vi "display loop.vi"(0 "display queues":T4, 1 "sample length":i32=5000, 2 "reset":bool, 3 "time range (s)":dbl=2.2 format="%#_13g", 4 "mag type":enum16{"absolute", "relative"}(ring), 5 "volt slope":bool, 7 "error in":errorcluster, 8 "trigger":bool, 9 "hysteresis":dbl=0.1 format="%#_13g", 10 "disk queues":T4, 12 "gain":dbl=1.0) -> (11 "voltage slope":dbl, 13 "slope graphs":cluster{dbl[], dbl[]}[](array[cluster]), 14 "lifetime":dbl, 16 "magnet vs time":cluster{dbl[], dbl[]}[](array[cluster]), 17 "mag pos axes limits":cluster{"mag pos max":dbl, "mag pos min":dbl}, 18 "voltage axes":T1, 19 "crossing stats":T2, 20 "fit parameters":cluster{"a":dbl, "b":dbl, "theta":dbl, "b0":dbl}, 21 "angle":dbl, 22 "deg/hr":dbl format="%0.2f", 23 "pulse statistics":T3, 24 "angle graph":cluster{dbl[], dbl[]}[](array[cluster]), 25 "voltage graphs":cluster{dbl[], dbl[]}[](array[cluster]), 26 "magnet graphs":T6(array[cluster]), 27 "error out":errorcluster)   [LabVIEW 2017]
uses:
  typedefs/queue cluster.ctl
  typedefs/reading queue.ctl
  typedefs/reading.ctl
  typedefs/readingType.ctl
  typedefs/reading1.ctl
panel:
  in  "hrs":bool=TRUE
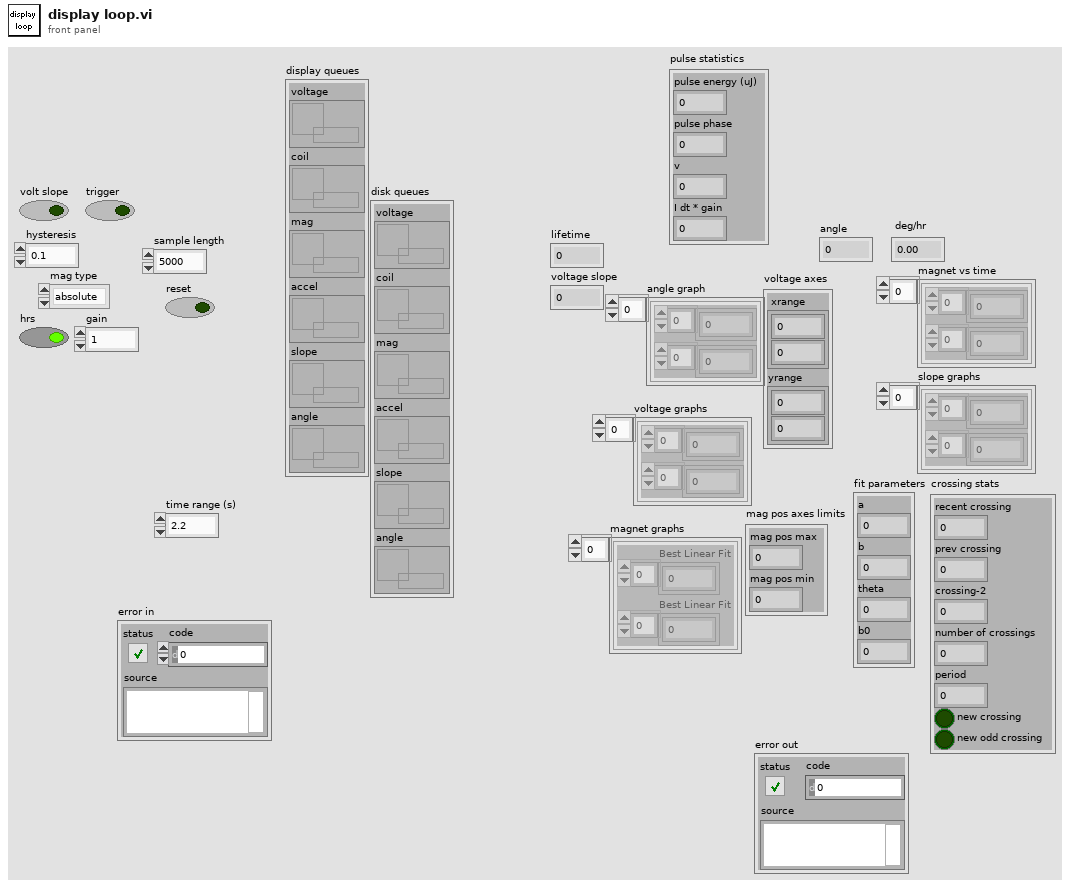
[diagram p1: front panel]
types:
  T1 = cluster{" xrange":cluster{dbl, dbl}, "yrange":cluster{dbl, dbl}}
  T2 = cluster{"recent crossing":dbl, "prev crossing":dbl, "crossing-2":dbl, "number of crossings":i32, "period":dbl, "new crossing":bool, "new odd crossing":bool}
  T3 = cluster{"pulse energy (uJ)":sgl, "pulse phase":dbl, "v":dbl, "I dt * gain":dbl}
  T4 = typedef "queue cluster.ctl" = cluster{"voltage":T5, "coil":T5, "mag":T5, "accel":T5, "slope":refnum<queue>, "angle":refnum<queue>}
  T5 = typedef "reading queue.ctl" = refnum<queue>
  T6 = cluster{"Best Linear Fit":dbl[], "Best Linear Fit":dbl[]}[]
  T7 = cluster{"time":dbl, "angle":dbl, "millisecond timer value":u32}
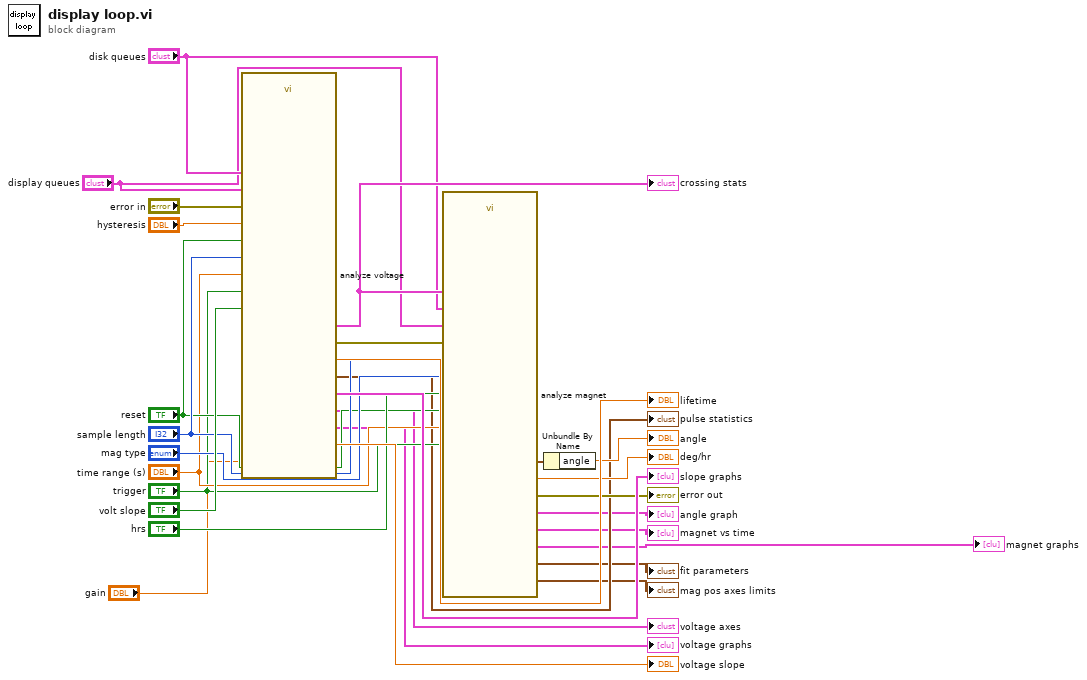
[diagram p0: block diagram]
diagram:
  n1 = call "analyze voltage.vi"("display queues"="display queues", "sample length"="sample length", "reset"="reset", "time range (s)"="time range (s)", "gain"="gain", "volt slope"="volt slope", "error in"="error in", "trigger"="trigger", "hysteresis"="hysteresis", "disk queues"="disk queues") -> ("crossing stats"=w23:T2, "lifetime"=→"lifetime":dbl, "voltage slope"=→"voltage slope":dbl, "voltage axes"=→"voltage axes":T1, "voltage graphs"=→"voltage graphs":cluster{dbl[], dbl[]}[], "slope graphs"=→"slope graphs":cluster{dbl[], dbl[]}[], "pulse statistics"=→"pulse statistics":T3, "error out"=w20:errorcluster)  [unwired: 10 in]
  "crossing stats" <- w23
  n2 = call "analyze magnet.vi"("display queues"="display queues", "disk queues"="disk queues", "trigger"="trigger", "graph type"="mag type", "error in (no error)"=w20, "reset"="reset", "fit length"="sample length", "hrs"="hrs", "toffset"="time range (s)", "crossing stats"=w23) -> ("mag pos axes limits"=→"mag pos axes limits":cluster{"mag pos max":dbl, "mag pos min":dbl}, "deg/hr"=→"deg/hr":dbl, "x-y magnet graph"=→"magnet graphs":cluster{sgl[], sgl[]}[], "magnet time graphs"=→"magnet vs time":cluster{dbl[], sgl[]}[], "fit parameters"=→"fit parameters":cluster{"a":dbl, "b":dbl, "theta":dbl, "b0":dbl}, "angle and time"=w11:T7, "angle graphs"=→"angle graph":cluster{dbl[], dbl[]}[], "error out"=→"error out":errorcluster)  [unwired: 2 in]
  n3 = Unbundle By Name(w11) -> ("angle"=→"angle":dbl)
